vi "HatchLatch_SLND.vi"(11 "Toggle?":bool) -> ()   [LabVIEW 2018]
uses:
  <vilib>/Rock Robotics/WPI/Solenoid/Deprecated/WPI_SolenoidSetBool.vi
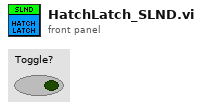
[diagram p1: front panel]
types:
  T1 = typedef "WPI_SolenoidDevRef.ctl" = cluster{"DevStatus":errorcluster, "Pneumatics Control Module":u8, "Forward Solenoid Channel":T2, "Reverse Solenoid Channel":T2}
  T2 = typedef "WPI_SolenoidChannel.ctl" = enum8{"Solenoid 0", "Solenoid 1", "Solenoid 2", "Solenoid 3", "Solenoid 4", "Solenoid 5", "Solenoid 6", "Solenoid 7", "Invalid"}
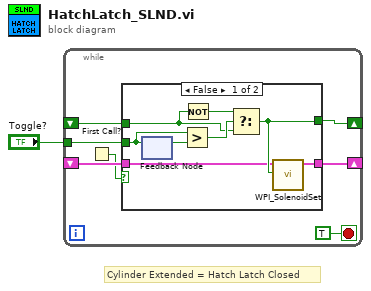
[diagram p0: block diagram]
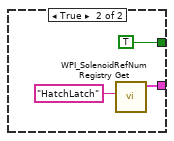
[diagram p2: hidden frame]
diagram:
  # "Cylinder Extended = Hatch Latch Closed"
  n1 = while {
    tunnel: "Toggle?" -> [w8]
    shift-right: [w5] -> _
    shift-left: _ -> [w6]
    shift-right: [w4] -> _
    shift-left: _ -> [w3]
    stop <- TRUE stop-if-true
    n2 = First Call?() -> (First Call?: T/F=w2:bool)
    n3 = case shown="False" w2 {
      tunnel: w8 -> [w15 _]
      tunnel: w6 -> [w13 _]
      tunnel: [w11 TRUE] -> w5
      tunnel: [w10 w19] -> w4
      tunnel: w3 -> [w9 _]
      frame False {
        n4 = feedback #1() -> (w16:bool)  [unwired: 1 in]
        n5 = feedback-in #1(w15) -> ()
        n6 = Greater?(x=w15, y=w16) -> (0:w14:bool)
        n7 = Not(x=w13) -> (.not. x?=w12:bool)
        n8 = Select(t=w12, s=w14, f=w13) -> (s? t:f=w11:bool)
        n9 = call-poly <vilib>:"WPI_SolenoidSet.vi"("Value"=w11, "SolenoidDevRef"=w9) -> ("SolenoidDevRef"=w10:T1)  [unwired: 8 in, 1 out]
      }
      frame True {
        n10 = call <vilib>:"WPI_SolenoidRefNum Registry Get.vi"("refnum name"="HatchLatch") -> ("SolenoidDevRef"=w19:T1)  [unwired: 9 in, 1 out]
      }
    }
  }
